vi "Galil_arrayDownloadFile.vi"() -> ()   [LabVIEW 2010]
panel:
  in  "Galil.IGalil":refnum<k7>
  out "Library Version:":string
  out "Response to LA command:":string
  out "error out":errorcluster
  out "Connected To:":string
  in  "Connection String:":string
  # "This vi Shows how to use the arrayDownloadFile function of the Galil Communications Library.  \n\nIf Connection String is left blank, the vi will open the connections dialog when run.  If a value is input into Connection String, the vi will attempt to connect to the controller at that address (ex COM1 19200).\n\nThe file \"array.csv\" contains 2 arrays - myArray[] and myArray2[].  This vi downloads the arrays in array.csv to the controller.  It then uploads myArray[] to array_1.csv and myArray2[] to array_2.csv.  Last it sends the LA command to the controller and displays the response."
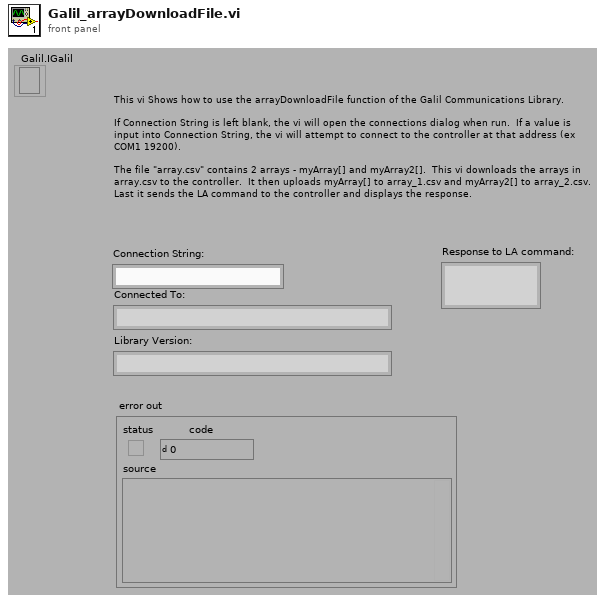
[diagram p1: front panel]
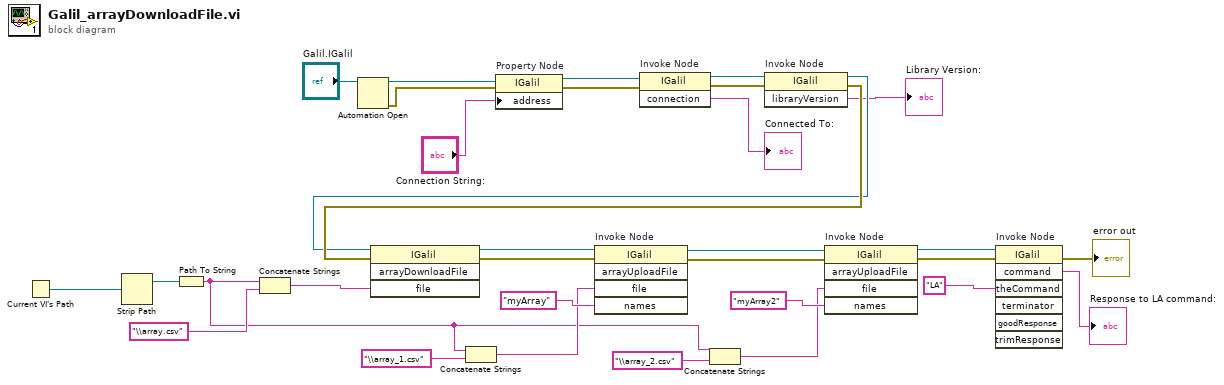
[diagram p0: block diagram]
diagram:
  n1 = Current VI's Path() -> (path=w9:path)
  n2 = Strip Path(path=w9) -> (stripped path=w8:path)  [unwired: 1 out]
  n3 = Path To String(path=w8) -> (string=w3:string)
  n4 = Concatenate Strings "Concatenate Strings"(w3, "\\array.csv") -> (w7:string)
  n5 = Automation Open(Automation Refnum="Galil.IGalil") -> (Automation Refnum=w32:refnum<k7>, error out=w30:errorcluster)  [unwired: 1 in, 2 out]
  n6 = Concatenate Strings "Concatenate Strings"(w3, "\\array_1.csv") -> (w5:string)
  n7 = property on="Property Node" class="IGalil"(reference=w32, error in=w30, "address"="Connection String:") -> (reference out=w31:refnum<k7>, error out=w29:errorcluster)
  n8 = invoke on="Invoke Node" class="IGalil" method="connection"(reference=w31, error in=w29) -> (reference out=w15:refnum<k7>, error out=w14:errorcluster, "connection"=→"Connected To:":string)  [unwired: 1 in]
  n9 = Concatenate Strings "Concatenate Strings"(w3, "\\array_2.csv") -> (w2:string)
  n10 = invoke on="Invoke Node" class="IGalil" method="libraryVersion"(reference=w15, error in=w14) -> (reference out=w12:refnum<k7>, error out=w13:errorcluster, "libraryVersion"=→"Library Version:":string)  [unwired: 1 in]
  n11 = invoke class="IGalil" method="arrayDownloadFile"(reference=w12, error in=w13, "file"=w7) -> (reference out=w22:refnum<k7>, error out=w21:errorcluster)  [unwired: 1 in, 2 out]
  n12 = invoke on="Invoke Node" class="IGalil" method="arrayUploadFile"(reference=w22, error in=w21, "file"=w5, "names"="myArray") -> (reference out=w24:refnum<k7>, error out=w23:errorcluster)  [unwired: 1 in, 3 out]
  n13 = invoke on="Invoke Node" class="IGalil" method="arrayUploadFile"(reference=w24, error in=w23, "file"=w2, "names"="myArray2") -> (reference out=w20:refnum<k7>, error out=w19:errorcluster)  [unwired: 1 in, 3 out]
  n14 = invoke on="Invoke Node" class="IGalil" method="command"(reference=w20, error in=w19, "theCommand"="LA") -> (error out=→"error out":errorcluster, "command"=→"Response to LA command:":string)  [unwired: 4 in, 5 out]
